vi "GitUpdateGitignore.vi"(8 "error in (no error)":errorcluster, 9 "Directory in":path, 11 "Git exec in":string) -> (0 "error out":errorcluster, 1 "Directory out":path, 3 "Git exec out":string)   [LabVIEW 2013]
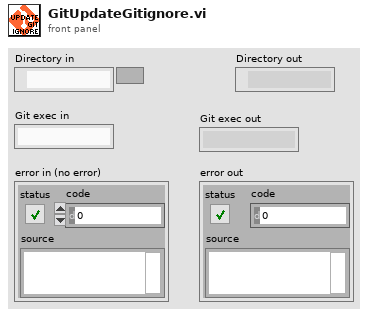
[diagram p1: front panel]
types:
  T1 = enum16{"open", "replace", "create", "open or create", "replace or create", "replace or create with confirmation"}
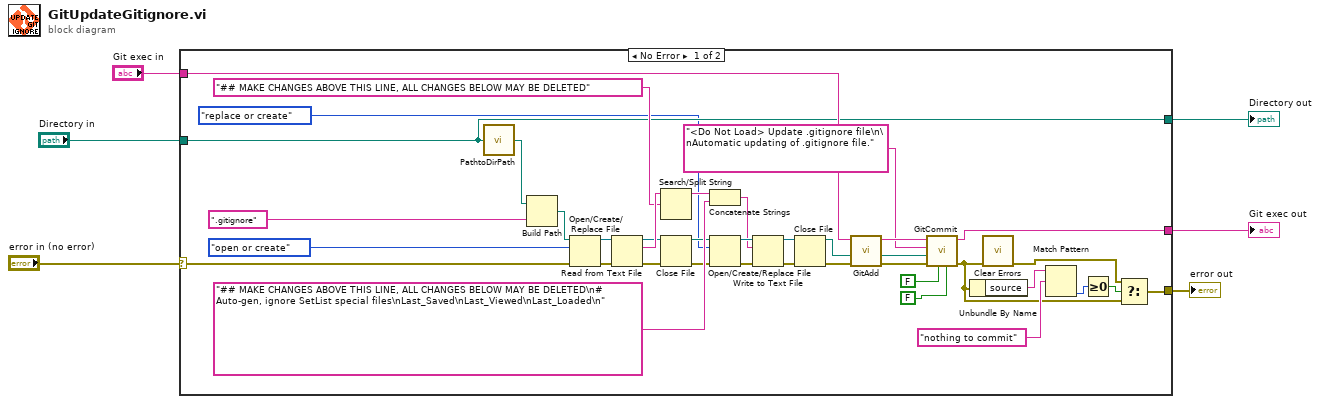
[diagram p0: block diagram]
diagram:
  n1 = case shown="No Error" "error in (no error)" {
    selector: "error in (no error)" -> [w26 w46]
    tunnel: "Git exec in" -> [w40 w47]
    tunnel: [w9 w46] -> w5
    tunnel: "Directory in" -> [w24 w48]
    tunnel: [w27 w47] -> w3
    tunnel: [w24 w48] -> w2
    frame No Error {
      n2 = call "PathtoDirPath.vi"("Path"=w24) -> ("Path out"=w25:path)
      n3 = Build Path(base path=w25, name or relative path=".gitignore") -> (appended path=w32:path)
      n4 = Open/Create/Replace File(file path (use dialog)=w32, error in=w26, operation (0:open)=T1."open or create") -> (refnum out=w44:refnum<file>, error out=w45:errorcluster)  [unwired: 3 in, 1 out]
      n5 = Read from Text File(file (use dialog)=w44, error in=w45) -> (refnum out=w22:refnum<file>, text=w43:string, error out=w23:errorcluster)  [unwired: 2 in, 1 out]
      n6 = Search/Split String(string=w43, search string/char (-)="## MAKE CHANGES ABOVE THIS LINE, ALL CHANGES BELOW MAY BE DELETED") -> (substring before match=w21:string)  [unwired: 1 in, 2 out]
      n7 = Close File(refnum=w22, error in=w23) -> (path=w19:path, error out=w18:errorcluster)
      n8 = Concatenate Strings(w21, "## MAKE CHANGES ABOVE THIS LINE, ALL CHANGES BELOW MAY BE DELETED\n# Auto-gen, ignore SetList special files\nLast_Saved\nLast_Viewed\nLast_Loaded\n" ("text")) -> (w14:string)
      n9 = Open/Create/Replace File(file path (use dialog)=w19, error in=w18, operation (0:open)=T1."replace or create") -> (refnum out=w17:refnum<file>, error out=w16:errorcluster)  [unwired: 3 in, 1 out]
      n10 = Write to Text File(file (use dialog)=w17, text=w14, error in=w16) -> (refnum out=w30:refnum<file>, error out=w29:errorcluster)  [unwired: 1 in, 1 out]
      n11 = Close File(refnum=w30, error in=w29) -> (path=w36:path, error out=w39:errorcluster)
      n12 = call "GitAdd.vi"("error in (no error)"=w39, "File"=w36, "Git exec"=w40) -> ("error out"=w38:errorcluster, "File out"=w37:path, "Git exec out"=w41:string)  [unwired: 5 in, 1 out]
      n13 = call "GitCommit.vi"("CommitAllAdded"=FALSE, "Allow Empty Commit?"=FALSE, "error in (no error)"=w38, "File"=w37, "Commit Message"="<Do Not Load> Update .gitignore file\n\nAutomatic updating of .gitignore file.", "Git exec"=w41) -> ("error out"=w8:errorcluster, "Git exec out"=w27:string)  [unwired: 2 in, 2 out]
      n14 = Unbundle By Name(w8) -> ("source"=w13:string)
      n15 = call <vilib>:"Clear Errors.vi"("error in (no error)"=w8) -> ("error out"=w7:errorcluster)  [unwired: 6 in]
      n16 = Match Pattern(string=w13, regular expression="nothing to commit") -> (offset past match=w11:i32)  [unwired: 1 in, 3 out]
      n17 = Greater Or Equal To 0?(x=w11) -> (x >= 0?=w10:bool)
      n18 = Select(t=w7, s=w10, f=w8) -> (s? t:f=w9:errorcluster)
    }
    frame Error {
    }
  }
  "error out" <- w5
  "Directory out" <- w2
  "Git exec out" <- w3
